vi "IF2_Clear_buffer.vi"(8 "error in (no error)":errorcluster, 11 "TCP Network Connection in":refnum<k5>) -> (0 "error out":errorcluster, 3 "TCP Network Connection out":refnum<k5>)   [LabVIEW 2015, in "IF2_Reader.lvlib"]
uses:
  IF2_Reader.lvlib
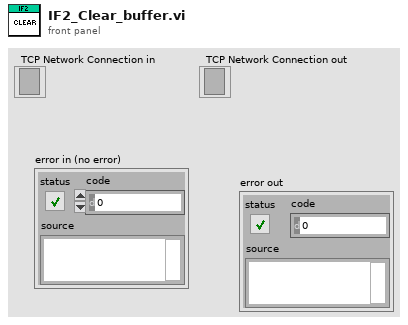
[diagram p1: front panel]
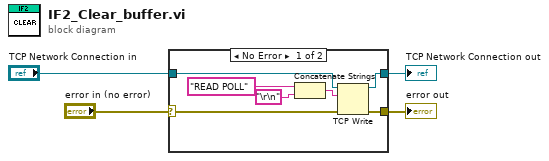
[diagram p0: block diagram]
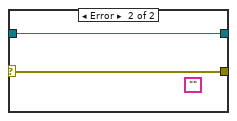
[diagram p2: hidden frame]
diagram:
  n1 = case shown="No Error" "error in (no error)" {
    selector: "error in (no error)" -> [w8 w12]
    tunnel: "TCP Network Connection in" -> [w7 w13]
    tunnel: [w6 w13] -> w3
    tunnel: [w5 w12] -> w1
    frame No Error {
      n2 = Concatenate Strings("READ POLL" ("data in"), "\r\n") -> (w9:string)
      n3 = TCP Write(connection ID=w7, data in=w9, error in (no error)=w8) -> (connection ID out=w6:refnum<k5>, error out=w5:errorcluster)  [unwired: 2 out]
    }
    frame Error {
      (unwired) ""
    }
  }
  "TCP Network Connection out" <- w3
  "error out" <- w1
